vi "cmd_set_feedback.vi"(8 "error in (no error)":errorcluster, 11 "JSON":string) -> (0 "error out":errorcluster)   [LabVIEW 2021]
doc: "Set feedback parameters\n \n :param feedback channels: Specifies the feedback channel 0 or 1\n :param Input channel: Specifies the input channel 0-7\n :param Output channel: Specifies the output channel 0-7\n :param Output imit (low): Specifies the lower output limit\n :param Output limit (high): Specifies the higher output limit\n :param Setpoint: Specifies the setpoint\n :param P gain: Specifies the propotional gain\n :param I gain: Specifies the integral gain\n :param Negative: if true, output value becomes negative\n :param Reset: reset the feedback\n :param Hold: hold the feedback\n :param Error limit (low): Specifies the lower error limit for wait for feedback\n :param Error limit (high): Specifies the higher error limit for wait for feedback\n :param wait for fb: Specifies the count for wait for weedback, if 0, wait for weedback is deactivated."
uses:
  fpga/fpga_feedback_config.ctl
  core/host_global_vars.vi
  <vilib>/Utility/error.llb/Error Cluster From Error Code.vi
  <vilib>/rvi/errors/niLvFpgaAdjustHostInterfaceError.vi
  <vilib>/rvi/interface/nirviReadWriteControl/nirviReadWriteControl.xnode
  FPGA Bitfiles/openlabspm_FPGATarget_fpgamain_eo-gUZR5D1g.lvbitx
  fpga/fpga_main.vi
  NiFpgaLv.dll
panel:
  in  "args":cluster{"fb config":T1, "fb channel":i32}
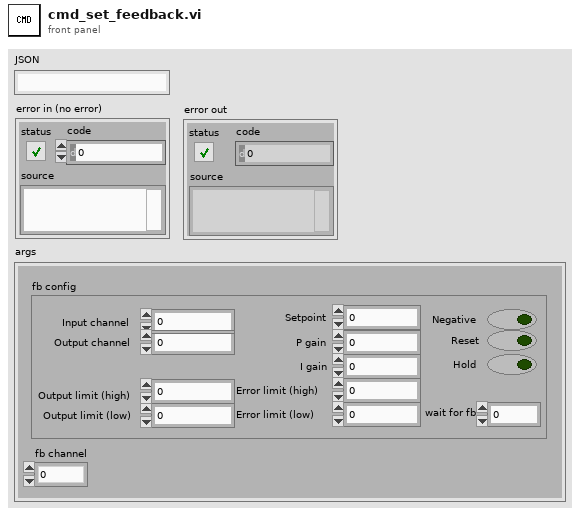
[diagram p1: front panel]
types:
  T1 = typedef "fpga_feedback_config.ctl" = cluster{"Setpoint":sgl, "Output limit (low)":sgl, "Output limit (high)":sgl, "P gain":sgl, "I gain":sgl, "Reset":bool, "Hold":bool, "Negative":bool, "Input channel":i16, "Output channel":i16, "wait for fb":i16, "Error limit (high)":sgl, "Error limit (low)":sgl}
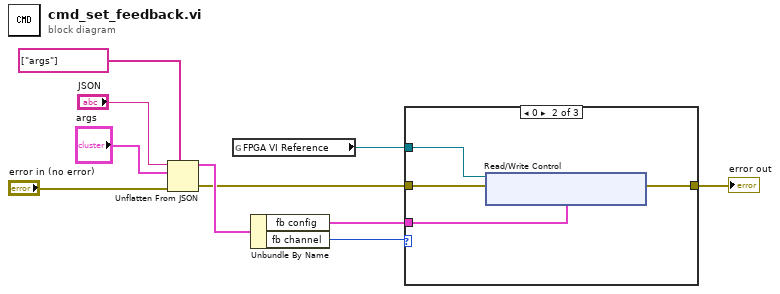
[diagram p0: block diagram]
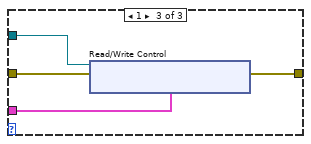
[diagram p3: hidden frame]
diagram:
  n1 = Unflatten From JSON(path=string[] ["args"], JSON string="JSON", type and defaults="args", error in (no error)="error in (no error)") -> (value=w6:cluster{"fb config":T1, "fb channel":i32}, error out=w4:errorcluster)  [unwired: 3 in]
  n2 = global read "host_global_vars.vi" "FPGA VI Reference"() -> (w7:refnum<k20>)
  n3 = Unbundle By Name(w6) -> ("fb config"=w5:T1, "fb channel"=w3:i32)
  n4 = case shown="0" w3 {
    tunnel: w7 -> [_ w15 w19]
    tunnel: w5 -> [_ w14 w18]
    tunnel: w4 -> [w11 w13 w17]
    tunnel: [w11 w12 w16] -> w2
    frame -1, Default {
    }
    frame 0 {
      n5 = xnode "Read/Write Control"("FPGA VI Reference In"=w15, "error in"=w13, "Feedback 0 config"=w14) -> ("error out"=w12:errorcluster)  [unwired: 1 out]
    }
    frame 1 {
      n6 = xnode "Read/Write Control"("FPGA VI Reference In"=w19, "error in"=w17, "Feedback 1 config"=w18) -> ("error out"=w16:errorcluster)  [unwired: 1 out]
    }
  }
  "error out" <- w2
